vi "LINC Get Item Properties.vi"(8 "error in (no error)":errorcluster, 11 "control reference":refnum<vi>) -> (0 "error out":errorcluster, 2 "properties":T1={"type"="", "bits"=-1, "elements"=0, "unit"="", "poly scale"=[], "ID"=FALSE, "REQUIRED"=FALSE})   [LabVIEW 2018, in "STEPkgDriver_LINC.lvlib"]
uses:
  STEPkgDriver_LINC.lvlib
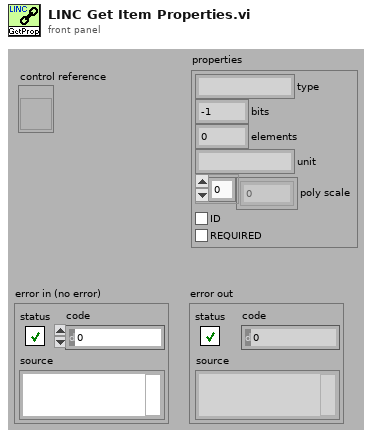
[diagram p1: front panel]
types:
  T1 = cluster{"type":string, "bits":i32, "elements":i32, "unit":string, "poly scale":dbl[], "ID":bool, "REQUIRED":bool}
  T2 = enum16{"Default", "TYPE=", "BITS=", "ELEMENTS=", "UNIT=", "CONV_POLY=", "ID", "REQUIRED"}
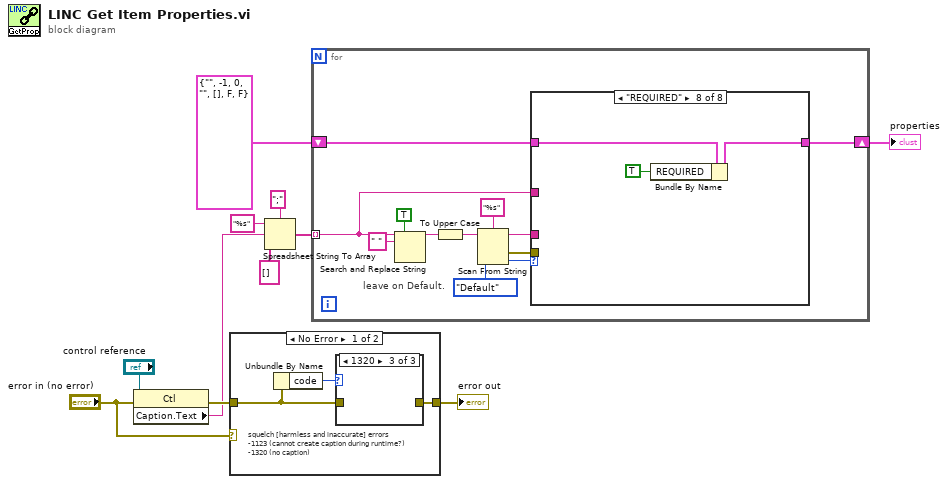
[diagram p0: block diagram]
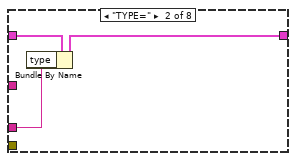
[diagram p6: hidden frame]
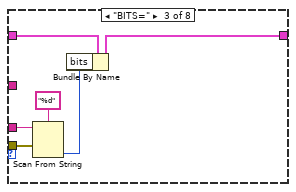
[diagram p7: hidden frame]
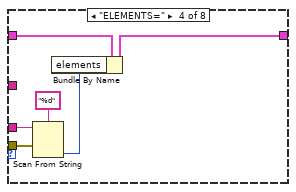
[diagram p8: hidden frame]
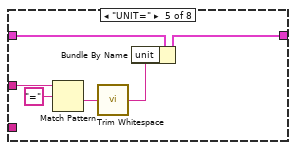
[diagram p9: hidden frame]
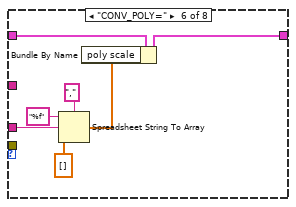
[diagram p10: hidden frame]
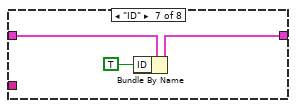
[diagram p11: hidden frame]
diagram:
  n1 = property class="Ctl"(reference="control reference", error in="error in (no error)") -> (error out=w5:errorcluster, "Caption.Text"=w2:string)  [unwired: 1 out]
  n2 = case shown="No Error" "error in (no error)" {
    tunnel: [w13 w16] -> w1
    tunnel: w5 -> [w12 w16]
    frame No Error {
      # "squelch [harmless and inaccurate] errors\n-1123 (cannot create caption during runtime?)\n-1320 (no caption)"
      n3 = Unbundle By Name(w12) -> ("code"=w14:i32)
      n4 = case shown="1320" w14 {
        tunnel: w12 -> [w15 _ _]
        tunnel: [w15 _ _] -> w13
        frame Default {
        }
        frame 1123 {
        }
        frame 1320 {
        }
      }
    }
    frame Error {
    }
  }
  "error out" <- w1
  n5 = Spreadsheet String To Array(delimiter (Tab)=";", format string="%s", spreadsheet string=w2, array type (2D Dbl)=string[] []) -> (array=w8:string[])
  n6 = for {
    tunnel: w8 -> [w19] mode=indexing
    shift-right: [w17] -> w7
    shift-left: T1 {"type"="", "bits"=-1, "elements"=0, "unit"="", "poly scale"=[], "ID"=FALSE, "REQUIRED"=FALSE} ("properties") -> [w18]
    # "leave on Default."
    n7 = Search and Replace String(replace all?=TRUE ("replace all? (F)"), input string=w19, search string=" ") -> (result string=w20:string)  [unwired: 5 in, 3 out]
    n8 = To Upper Case(1:w20) -> (0:w27:string)
    n9 = Scan From String(format string="%s", input string=w27, default 1=T2."Default") -> (remaining string=w24:string, error out=w23:errorcluster, output 1=w25:T2)  [unwired: 2 in, 1 out]
    n10 = case shown="\"REQUIRED\"" w25 {
      tunnel: w24 -> [_ w30 w37 w43 _ w54 _ _]
      tunnel: w23 -> [_ _ w36 w42 _ _ _ _]
      tunnel: w19 -> [_ _ _ _ w50 _ _ _]
      tunnel: w18 -> [w29 w32 w35 w41 w47 w53 w60 w63]
      tunnel: [w29 w31 w34 w40 w46 w52 w59 w62] -> w17
      frame "Default" {
      }
      frame "TYPE=" {
        n11 = Bundle By Name(cluster=w32, "type"=w30) -> (w31:T1)
      }
      frame "BITS=" {
        n12 = Scan From String(format string="%d", input string=w37, error in=w36) -> (output 1=w33:i32)  [unwired: 2 in, 3 out]
        n13 = Bundle By Name(cluster=w35, "bits"=w33) -> (w34:T1)
      }
      frame "ELEMENTS=" {
        n14 = Scan From String(format string="%d", input string=w43, error in=w42) -> (output 1=w39:i32)  [unwired: 2 in, 3 out]
        n15 = Bundle By Name(cluster=w41, "elements"=w39) -> (w40:T1)
      }
      frame "UNIT=" {
        n16 = Match Pattern(string=w50, regular expression="=" ("search string/char (-)")) -> (after substring=w48:string)  [unwired: 1 in, 3 out]
        n17 = call <vilib>:"Trim Whitespace.vi"("string"=w48) -> ("trimmed string"=w45:string)  [unwired: 1 in]
        n18 = Bundle By Name(cluster=w47, "unit"=w45) -> (w46:T1)
      }
      frame "CONV_POLY=" {
        n19 = Spreadsheet String To Array(delimiter (Tab)=",", format string="%f", spreadsheet string=w54, array type (2D Dbl)=dbl[] []) -> (array=w51:dbl[])
        n20 = Bundle By Name(cluster=w53, "poly scale"=w51) -> (w52:T1)
      }
      frame "ID" {
        n21 = Bundle By Name(cluster=w60, "ID"=TRUE) -> (w59:T1)
      }
      frame "REQUIRED" {
        n22 = Bundle By Name(cluster=w63, "REQUIRED"=TRUE ("ID")) -> (w62:T1)
      }
    }
  }
  "properties" <- w7
